vi "login panel.vi"() -> ()   [LabVIEW 2019]
uses:
  Control 1.ctl
panel:
  in  "submit":T1
  in  "password":string
  in  "username":string
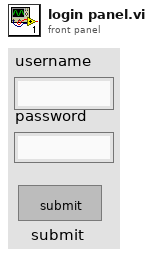
[diagram p1: front panel]
types:
  T1 = typedef "Control 1.ctl" = bool
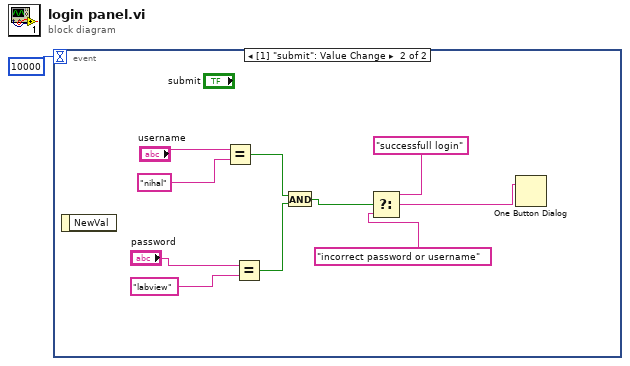
[diagram p0: block diagram]
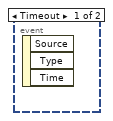
[diagram p2: hidden frame]
diagram:
  n1 = event shown="[1] \"submit\": Value Change" {
    selector: _ -> [_ _]
    dyn-events: _ -> [_ _]
    timeout: 10000 -> [_ _]
    event Timeout {
      n2 = event-data() -> ()  [unwired: 1 in, 3 out]
    }
    event Value Change {
      n3 = event-data() -> ()  [unwired: 1 in, 1 out]
      n4 = Equal?(x="username", y="nihal") -> (x = y?=w8:bool)
      n5 = Equal?(x="password", y="labview") -> (x = y?=w7:bool)
      n6 = And(x=w8, y=w7) -> (x .and. y?=w6:bool)
      n7 = Select(t="successfull login", s=w6, f="incorrect password or username") -> (s? t:f=w3:string)
      n8 = One Button Dialog(message=w3) -> ()  [unwired: 1 in, 1 out]
    }
  }
